vi "Write Other Images.vi"(8 "error in (no error)":errorcluster, 10 "Other Images":refnum<class "SVGImage.lvclass">[](array[class]), 11 "ParseVectorFile in":refnum<class "ParseVectorFile.lvclass">) -> (0 "error out":errorcluster, 3 "ParseVectorFile out":refnum<class "ParseVectorFile.lvclass">)   [LabVIEW 2019, in "ParseVectorFile.lvclass"]
uses:
  ParseVectorFile.lvclass
  Image/SVGImage.lvclass
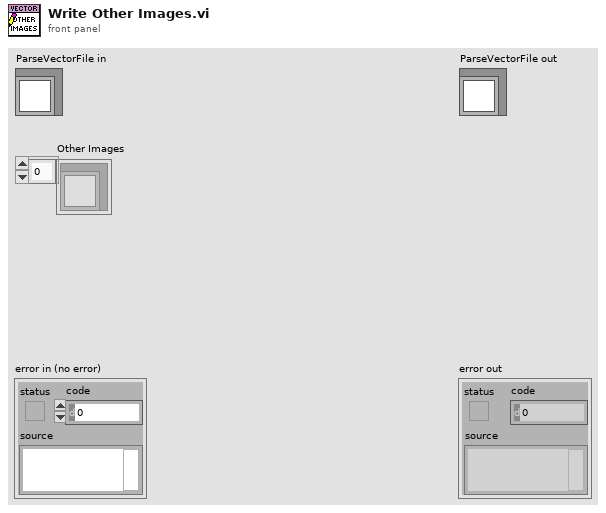
[diagram p1: front panel]
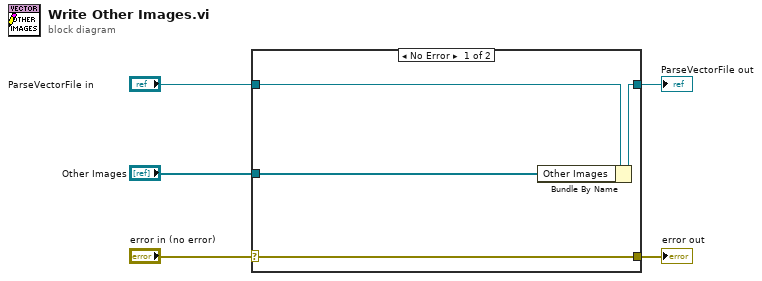
[diagram p0: block diagram]
diagram:
  n1 = case shown="No Error" "error in (no error)" {
    selector: "error in (no error)" -> [w9 w10]
    tunnel: [w9 w10] -> w4
    tunnel: [w7 w11] -> w2
    tunnel: "ParseVectorFile in" -> [w8 w11]
    tunnel: "Other Images" -> [w6 _]
    frame No Error {
      n2 = Bundle By Name(cluster=w8, "Other Images"=w6) -> (w7:refnum<class "ParseVectorFile.lvclass">)
    }
    frame Error {
    }
  }
  "error out" <- w4
  "ParseVectorFile out" <- w2
